vi "GEA2 Message Sent Event Handler.vi"(4 "Send Data":refnum<user-event>, 5 "Event Data":T1, 6 "Control Ref":refnum<k24>, 7 "Event Common Data":T2) -> ()   [LabVIEW 2023, in "GEA2_Toolkit.lvlib"]
uses:
  library/GEA2_Toolkit.lvlib
  D:/Common/LabVIEW GEA2 Toolkit/source/GEA3 DLL Source/GeaCommunication.dll
  source/GEA3 DLL Source/GeaCommunication.dll
  type defs/Data Out.ctl
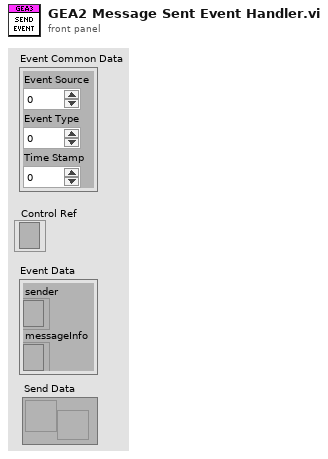
[diagram p1: front panel]
types:
  T1 = cluster{"sender":refnum<k24>, "messageInfo":refnum<k24>}
  T2 = cluster{"Event Source":i32, "Event Type":u32, "Time Stamp":u32}
  T3 = typedef "GEA2_Toolkit.lvlib/Data Out.ctl" = cluster{"Source":u8, "Destination":u8, "Command":u8, "Length":u8, "CRC":u16, "Message":string}
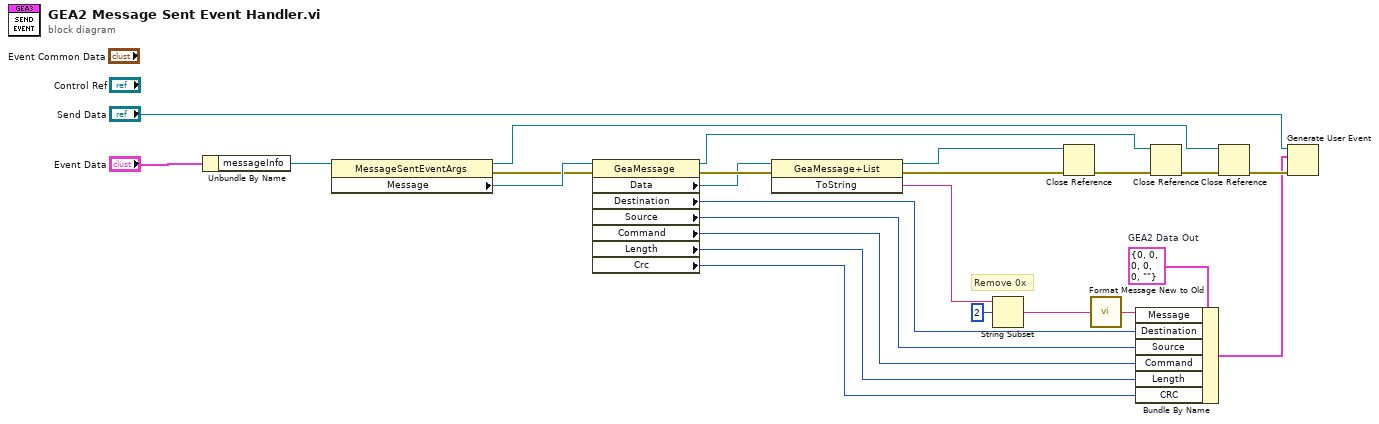
[diagram p0: block diagram]
diagram:
  w1 = T3 {"Source"=0, "Destination"=0, "Command"=0, "Length"=0, "CRC"=0, "Message"=""}  # GEA2 Data Out
  # "Remove 0x"
  n1 = Unbundle By Name("Event Data") -> ("messageInfo"=w25:refnum<k24>)
  n2 = property class="MessageSentEventArgs"(reference=w25) -> (reference out=w9:refnum<k24>, error out=w17:errorcluster, "Message"=w23:refnum<k24>)  [unwired: 1 in]
  n3 = property class="GeaMessage"(reference=w23, error in=w17) -> (reference out=w10:refnum<k24>, error out=w13:errorcluster, "Data"=w8:refnum<k24>, "Destination"=w22:u8, "Source"=w21:u8, "Command"=w20:u8, "Length"=w19:u8, "Crc"=w18:u16)
  n4 = invoke class="GeaMessage+List" method="ToString"(reference=w8, error in=w13) -> (reference out=w11:refnum<k24>, error out=w12:errorcluster, "ToString"=w7:string)  [unwired: 1 in]
  n5 = String Subset(string=w7, offset (0)=2) -> (substring=w5:string)  [unwired: 1 in]
  n6 = Close Reference(reference=w11, error in (no error)=w12) -> (error out=w24:errorcluster)
  n7 = call "Format Message New to Old.vi"("Raw Message In"=w5) -> ("Conv Message Out"=w14:string)  [unwired: 14 in]
  n8 = Bundle By Name(cluster=w1, "Message"=w14, "Destination"=w22, "Source"=w21, "Command"=w20, "Length"=w19, "CRC"=w18) -> (w2:T3)
  n9 = Close Reference(reference=w10, error in (no error)=w24) -> (error out=w16:errorcluster)
  n10 = Close Reference(reference=w9, error in (no error)=w16) -> (error out=w15:errorcluster)
  n11 = Generate User Event(user event="Send Data", event data cluster=w2, error in=w15) -> ()  [unwired: 1 in, 2 out]
